vi "Gen Info Data from INI.vi"(8 "error in":errorcluster, 11 "Config Refnum in":T1) -> (0 "error out":errorcluster, 3 "Config Refnum out":T1, 4 "Generator_Info":T2)   [LabVIEW 2018]
uses:
  <vilib>/Utility/config.llb/Config Data RefNum.ctl
  <vilib>/ORNL/CSEISMIC DDS/CSEISMIC DDS Base/Data Types/Generator_Info.ctl
  <vilib>/ORNL/CSEISMIC DDS/CSEISMIC DDS Base/Data Types/Controls/DeviceID.ctl
  <vilib>/ORNL/CSEISMIC DDS/CSEISMIC DDS Base/Data Types/Controls/EfficiencyCurve.ctl
  <vilib>/Utility/config.llb/Read Key (String).vi
  <vilib>/Utility/config.llb/Read Key (Double).vi
  <vilib>/Utility/config.llb/NI_LVConfig.lvlib
  <vilib>/ORNL/CSEISMIC DDS/CSEISMIC DDS Base/CSEISMIC DDS.lvclass
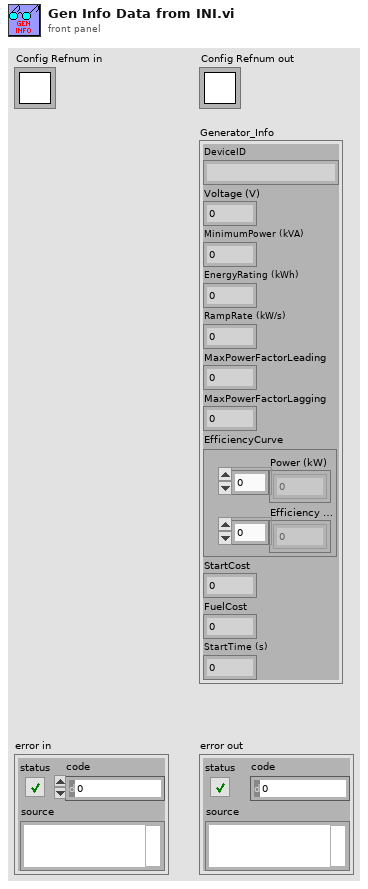
[diagram p1: front panel]
types:
  T1 = typedef "NI_LVConfig.lvlib/Config Data RefNum.ctl" = refnum<k1>
  T2 = typedef "CSEISMIC DDS.lvlib/CSEISMIC DDS.lvclass/Generator_Info.ctl" = cluster{"DeviceID":T3, "Voltage (V)":dbl, "MinimumPower (kVA)":dbl, "EnergyRating (kWh)":dbl, "RampRate (kW/s)":dbl, "MaxPowerFactorLeading":dbl, "MaxPowerFactorLagging":dbl, "EfficiencyCurve":T4, "StartCost":dbl, "FuelCost":dbl, "StartTime (s)":dbl}
  T3 = typedef "CSEISMIC DDS.lvlib/CSEISMIC DDS.lvclass/DeviceID.ctl" = string
  T4 = typedef "CSEISMIC DDS.lvlib/CSEISMIC DDS.lvclass/EfficiencyCurve.ctl" = cluster{"Power (kW)":dbl[], "Efficiency (%)":dbl[]}
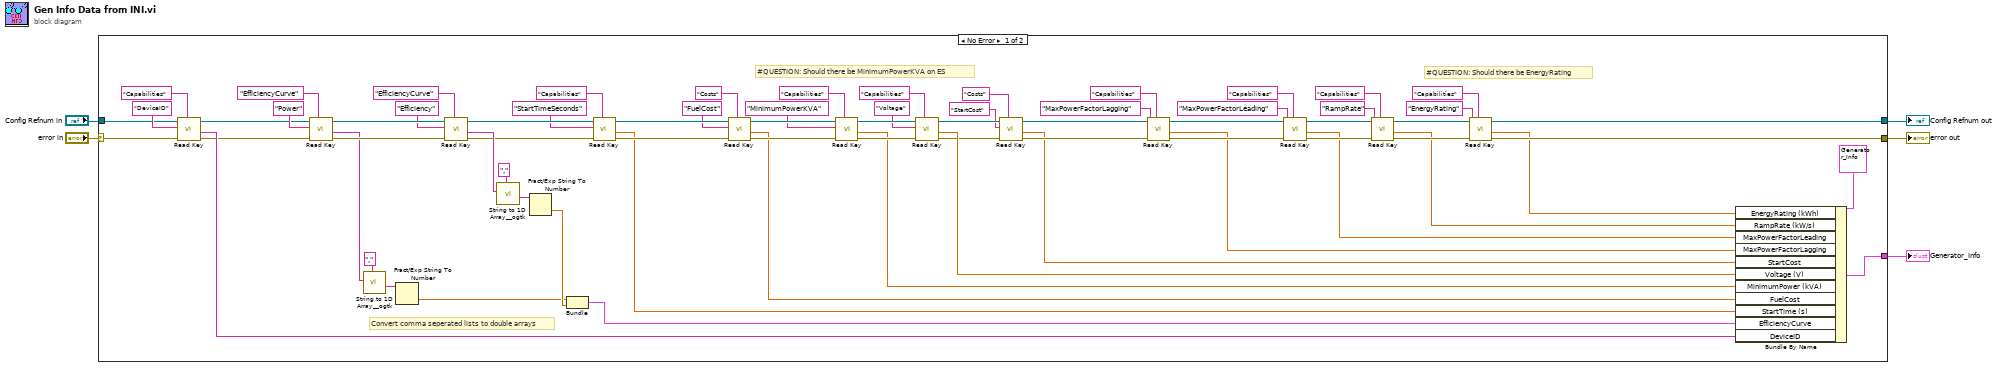
[diagram p0: block diagram]
diagram:
  n1 = case shown="No Error" "error in" {
    selector: "error in" -> [w18 w78]
    tunnel: [w76 w78] -> w5
    tunnel: [w72 w77] -> w4
    tunnel: [w68 _] -> w3
    tunnel: "Config Refnum in" -> [w19 w77]
    frame No Error {
      # "#QUESTION: Should there be MinimumPowerKVA on ES"
      # "#QUESTION: Should there be EnergyRating"
      # "Convert comma seperated lists to double arrays"
      n2 = call-poly <vilib>:"Read Key.vi"("section"="Capabilities", "error in (no error)"=w18, "key"="DeviceID", "refnum"=w19) -> ("error out"=w20:errorcluster, "value"=w24:string, "refnum out"=w21:T1)  [unwired: 4 in, 1 out]
      n3 = call-poly <vilib>:"Read Key.vi"("section"="EfficiencyCurve", "error in (no error)"=w20, "key"="Power", "refnum"=w21) -> ("error out"=w34:errorcluster, "value"=w27:string, "refnum out"=w33:T1)  [unwired: 4 in, 1 out]
      n4 = call <userlib>:"String to 1D Array__ogtk.vi"("delimiter (Tab)"=",", "string"=w27) -> ("Array of Strings"=w29:string[])  [unwired: 9 in]
      n5 = Fract/Exp String To Number(string=w29) -> (number=w54:dbl[])  [unwired: 3 in, 1 out]
      n6 = call-poly <vilib>:"Read Key.vi"("section"="EfficiencyCurve", "error in (no error)"=w34, "key"="Efficiency", "refnum"=w33) -> ("error out"=w38:errorcluster, "value"=w45:string, "refnum out"=w37:T1)  [unwired: 4 in, 1 out]
      n7 = call <userlib>:"String to 1D Array__ogtk.vi"("delimiter (Tab)"=",", "string"=w45) -> ("Array of Strings"=w43:string[])  [unwired: 9 in]
      n8 = Fract/Exp String To Number(string=w43) -> (number=w55:dbl[])  [unwired: 3 in, 1 out]
      n9 = Bundle(w54, w55) -> (w17:cluster{dbl[], dbl[]})  [unwired: 1 in]
      n10 = call-poly <vilib>:"Read Key.vi"("section"="Capabilities", "error in (no error)"=w38, "key"="StartTimeSeconds", "refnum"=w37) -> ("error out"=w41:errorcluster, "value"=w16:dbl, "refnum out"=w42:T1)  [unwired: 4 in, 1 out]
      n11 = call-poly <vilib>:"Read Key.vi"("section"="Costs", "error in (no error)"=w41, "key"="FuelCost", "refnum"=w42) -> ("error out"=w51:errorcluster, "value"=w15:dbl, "refnum out"=w50:T1)  [unwired: 4 in, 1 out]
      n12 = call-poly <vilib>:"Read Key.vi"("section"="Capabilities", "error in (no error)"=w51, "key"="MinimumPowerKVA", "refnum"=w50) -> ("error out"=w53:errorcluster, "value"=w13:dbl, "refnum out"=w52:T1)  [unwired: 4 in, 1 out]
      n13 = call-poly <vilib>:"Read Key.vi"("section"="Capabilities", "error in (no error)"=w53, "key"="Voltage", "refnum"=w52) -> ("error out"=w10:errorcluster, "value"=w14:dbl, "refnum out"=w12:T1)  [unwired: 4 in, 1 out]
      n14 = call-poly <vilib>:"Read Key.vi"("section"="Costs", "error in (no error)"=w10, "key"="StartCost", "refnum"=w12) -> ("error out"=w9:errorcluster, "value"=w6:dbl, "refnum out"=w11:T1)  [unwired: 4 in, 1 out]
      n15 = call-poly <vilib>:"Read Key.vi"("section"="Capabilities", "error in (no error)"=w9, "key"="MaxPowerFactorLagging", "refnum"=w11) -> ("error out"=w73:errorcluster, "value"=w64:dbl, "refnum out"=w69:T1)  [unwired: 4 in, 1 out]
      n16 = call-poly <vilib>:"Read Key.vi"("section"="Capabilities", "error in (no error)"=w73, "key"="MaxPowerFactorLeading", "refnum"=w69) -> ("error out"=w74:errorcluster, "value"=w65:dbl, "refnum out"=w70:T1)  [unwired: 4 in, 1 out]
      n17 = call-poly <vilib>:"Read Key.vi"("section"="Capabilities", "error in (no error)"=w74, "key"="RampRate", "refnum"=w70) -> ("error out"=w75:errorcluster, "value"=w66:dbl, "refnum out"=w71:T1)  [unwired: 4 in, 1 out]
      n18 = call-poly <vilib>:"Read Key.vi"("section"="Capabilities", "error in (no error)"=w75, "key"="EnergyRating", "refnum"=w71) -> ("error out"=w76:errorcluster, "value"=w67:dbl, "refnum out"=w72:T1)  [unwired: 4 in, 1 out]
      n19 = Bundle By Name(cluster=T2 {"DeviceID"="", "Voltage (V)"=0.0, "MinimumPower (kVA)"=0.0, "EnergyRating (kWh)"=0.0, "RampRate (kW/s)"=0.0, "MaxPowerFactorLeading"=0.0, "MaxPowerFactorLagging"=0.0, "EfficiencyCurve"={"Power (kW)"=[], "Efficiency (%)"=[]}, "StartCost"=0.0, "FuelCost"=0.0, "StartTime (s)"=0.0} ("Generator_Info"), "EnergyRating (kWh)"=w67, "RampRate (kW/s)"=w66, "MaxPowerFactorLeading"=w65, "MaxPowerFactorLagging"=w64, "StartCost"=w6, "Voltage (V)"=w14, "MinimumPower (kVA)"=w13, "FuelCost"=w15, "StartTime (s)"=w16, "EfficiencyCurve"=w17, "DeviceID"=w24) -> (w68:T2)
    }
    frame Error {
    }
  }
  "error out" <- w5
  "Config Refnum out" <- w4
  "Generator_Info" <- w3
